vi "LETRAS.vi"(8 "error in (no error)":errorcluster, 11 "IMAGE in":T1) -> (0 "error out":errorcluster, 2 "String (OCR/OCV 1)":string)   [LabVIEW 2020, in "Analisis.lvlib"]
uses:
  Analisis.lvlib
  <vilib>/vision/Image Controls.llb/IMAQ Image.ctl
  <vilib>/vision/NI_Vision_Development_Module.lvlib
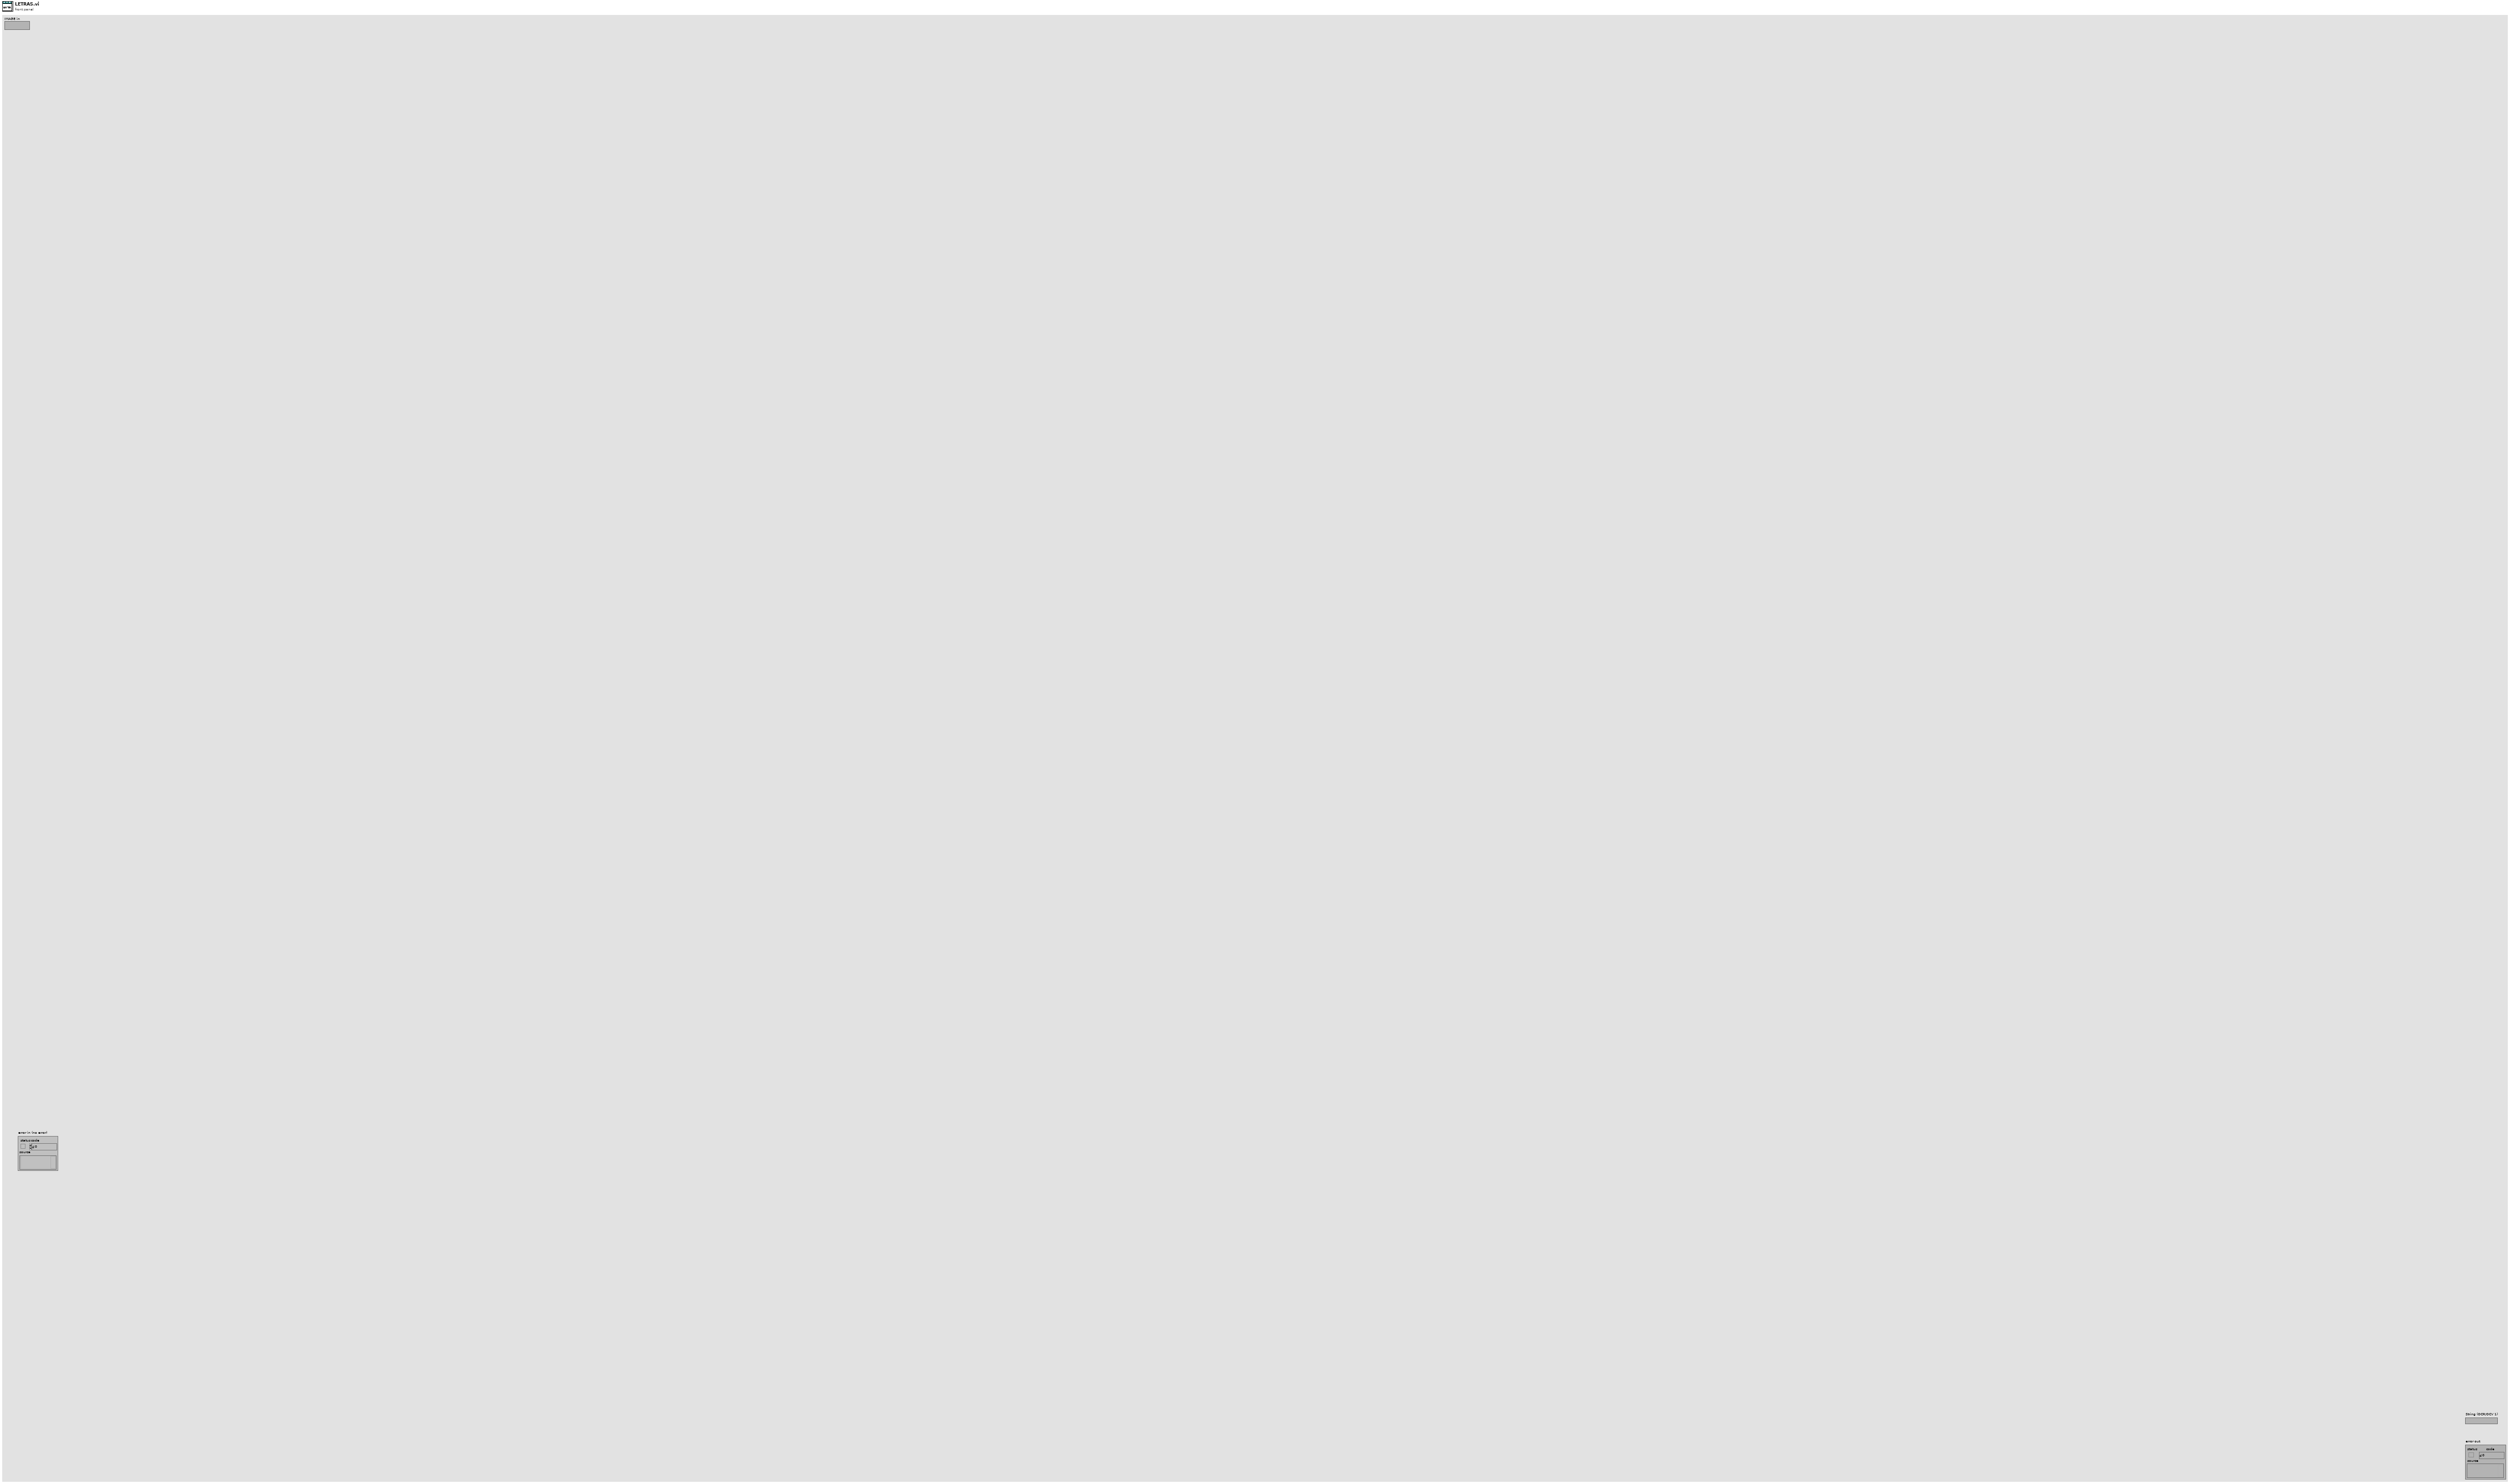
[diagram p1: front panel]
types:
  T1 = typedef "IMAQ Image.ctl" = refnum<image>
  T2 = cluster{"Threshold Data":cluster{"Method":enum16{"Fixed Range", "Uniform", "Linear", "Non Linear", "Local", "Color"}, "Looking for":u32, "Color Mode":u32, "Kernel Size":cluster{"Width":i32, "Height":i32}, "Ranges":cluster{"Min":i32, "Max":i32}[]}, "Reject Border":bool, "Number Of Erosions":i32, "Size & Spacing":cluster{"Segment Algorithm":u16, "Min Bounding Rect Width":i32, "Max Bounding Rect Width":i32, "Min Bounding Rect Height":i32, "Max Bounding Rect Height":i32, "Min Character Size":i32, "Max Character Size":i32, "Min Char Spacing":i32, "Max Horiz Element Spacing":i32, "Max Vert Element Spacing":i32, "Max Space Distance":i32}, "Read Options":cluster{"Read Strategy":i32, "Read Resolution":i32, "Scale Dependant":bool, "Aspect Ratio":i32, "Acceptance Level":i32, "Substitution Character":string, "MultiLine":bool}, "Valid Characters":cluster{"Pre-defined characters":i32, "User-defined characters":string}[], "Use Text Pattern":bool, "Orientation":u32, "# Lines Expected":u32, "Number of Blocks":i32}
  T3 = cluster{"Global Rectangle":i32[], "Contours":cluster{"ID":enum32{"External", "Internal"}, "Type":u32, "Coordinates":i32[]}[]}
  T4 = typedef "IMAQ OCR Session.ctl" = refnum<k1>
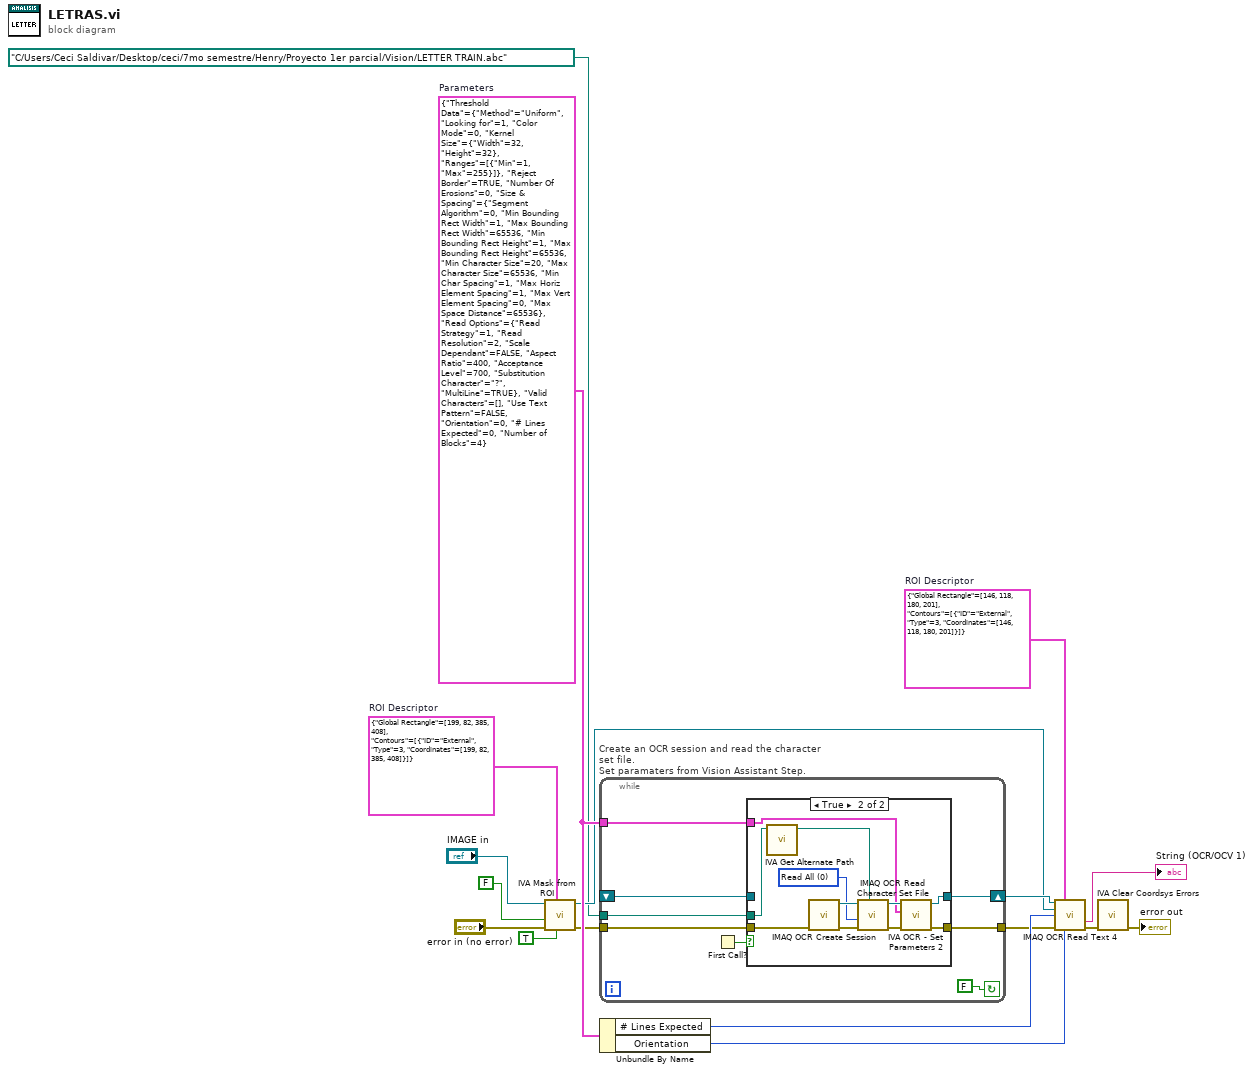
[diagram p0: block diagram]
diagram:
  w11 = T2 {"Threshold Data"={"Method"=enum."Uniform", "Looking for"=1, "Color Mode"=0, "Kernel Size"={"Width"=32, "Height"=32}, "Ranges"=[{"Min"=1, "Max"=255}]}, "Reject Border"=TRUE, "Number Of Erosions"=0, "Size & Spacing"={"Segment Algorithm"=0, "Min Bounding Rect Width"=1, "Max Bounding Rect Width"=65536, "Min Bounding Rect Height"=1, "Max Bounding Rect Height"=65536, "Min Character Size"=20, "Max Character Size"=65536, "Min Char Spacing"=1, "Max Horiz Element Spacing"=1, "Max Vert Element Spacing"=0, "Max Space Distance"=65536}, "Read Options"={"Read Strategy"=1, "Read Resolution"=2, "Scale Dependant"=FALSE, "Aspect Ratio"=400, "Acceptance Level"=700, "Substitution Character"="?", "MultiLine"=TRUE}, "Valid Characters"=[], "Use Text Pattern"=FALSE, "Orientation"=0, "# Lines Expected"=0, "Number of Blocks"=4}  # Parameters
  w9 = T3 {"Global Rectangle"=[146, 118, 180, 201], "Contours"=[{"ID"=enum."External", "Type"=3, "Coordinates"=[146, 118, 180, 201]}]}  # ROI Descriptor
  w2 = T3 {"Global Rectangle"=[199, 82, 385, 408], "Contours"=[{"ID"=enum."External", "Type"=3, "Coordinates"=[199, 82, 385, 408]}]}  # ROI Descriptor
  n1 = call <vilib>:"IVA Mask from ROI.vi"("Shrink"=TRUE, "ROI Descriptor"=w2, "error in (no error)"="error in (no error)", "Out / In"=FALSE, "Image Src"="IMAGE in") -> ("error out"=w6:errorcluster, "Image Out"=w10:T1)  [unwired: 5 out]
  n2 = while "Create an OCR session and read the character set file.\nSet paramaters from Vision Assistant Step." {
    shift-right: [w22] -> w13
    shift-left: _ -> [w21]
    tunnel: w6 -> [w24]
    tunnel: w11 -> [w20]
    tunnel: path "C:/Users/Ceci Saldivar/Desktop/ceci/7mo semestre/Henry/Proyecto 1er parcial/Vision/LETTER TRAIN.abc" ("File Path") -> [w19]
    tunnel: [w18] -> w12
    stop <- FALSE continue-if-true
    n3 = First Call?() -> (First Call?: T/F=w23:bool)
    n4 = case shown="True" w23 {
      tunnel: w19 -> [_ w31]
      tunnel: w24 -> [w26 w35]
      tunnel: [w27 w33] -> w22
      tunnel: [w26 w32] -> w18
      tunnel: w20 -> [_ w28]
      tunnel: w21 -> [w27 _]
      frame False {
      }
      frame True {
        w36 = 0 items=["Read All", "Read Character Set Only", "Read Properties Only"] ("Read Options")
        n5 = call <vilib>:"IVA Get Alternate Path.vi"("Path In"=w31) -> ("Path Out"=w30:path)  [unwired: 10 out]
        n6 = call "IMAQ OCR Create Session"("error in (no error)"=w35) -> ("error out"=w37:errorcluster, "IMAQ OCR Session"=w38:T4)  [unwired: 9 out]
        n7 = call "IMAQ OCR Read Character Set File"("File Path"=w30, "error in (no error)"=w37, "Read Options"=w36, "IMAQ OCR Session"=w38) -> ("error out"=w34:errorcluster, "IMAQ OCR Session (dup)"=w29:T4)  [unwired: 1 in, 5 out]
        n8 = call <vilib>:"IVA OCR - Set Parameters 2.vi"("error in (no error)"=w34, "Parameters"=w28, "IMAQ OCR Session"=w29) -> ("error out"=w32:errorcluster, "IMAQ OCR Session Out"=w33:T4)  [unwired: 7 in]
      }
    }
  }
  n9 = Unbundle By Name(w11) -> ("# Lines Expected"=w15:u32, "Orientation"=w14:u32)
  n10 = call "IMAQ OCR Read Text 4"("IMAQ OCR Session"=w13, "ROI Descriptor"=w9, "Image"=w10, "Number of Lines Requested"=w15, "error in (no error)"=w12, "Orientation"=w14) -> ("Read String"=→"String (OCR/OCV 1)":string, "error out"=w16:errorcluster)  [unwired: 8 out]
  n11 = call <vilib>:"IVA Clear Coordsys Errors.vi"("error in (no error)"=w16) -> ("error out"=→"error out":errorcluster)  [unwired: 10 in]
